vi "Default SubVIs.vi"(8 "error in (no error)":errorcluster, 10 "Unbundler Terminals":refnum<vi>[](array[refnum]), 11 "VI in":refnum<vi>) -> (0 "error out":errorcluster, 2 "SubVI Outputs":refnum<vi>[](array[refnum]), 3 "VI":refnum<vi>)   [LabVIEW 2020, in "Conditum-Tools.lvlib" / "Entity Editor.lvclass"]
uses:
  Entity Editor.lvclass
  <vilib>/Utility/traverseref.llb/TRef TravTarget.ctl
  <vilib>/Utility/miscctls.llb/LVPositionTypeDef.ctl
  <vilib>/IlluminatedG/IG Conditum Base/Conditum/Columns/Type/Set Default.vi
  <vilib>/Utility/traverseref.llb/VI Scripting - Traverse.lvlib
  <vilib>/IlluminatedG/IG Conditum Base/Conditum/Columns/Type/Type.lvclass
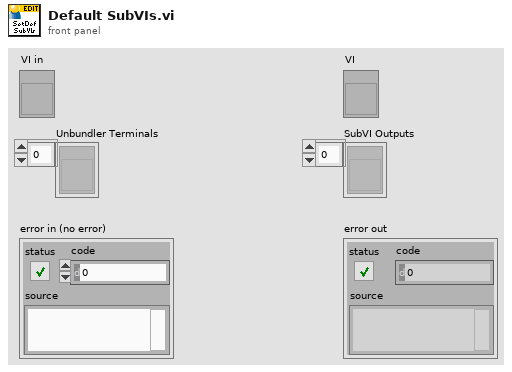
[diagram p1: front panel]
types:
  T1 = typedef "LVPositionTypeDef.ctl" = cluster{"Left":i32, "Top":i32}
  T2 = typedef "TRef TravTarget.ctl" = enum16{"FP", "BD", "Other"}
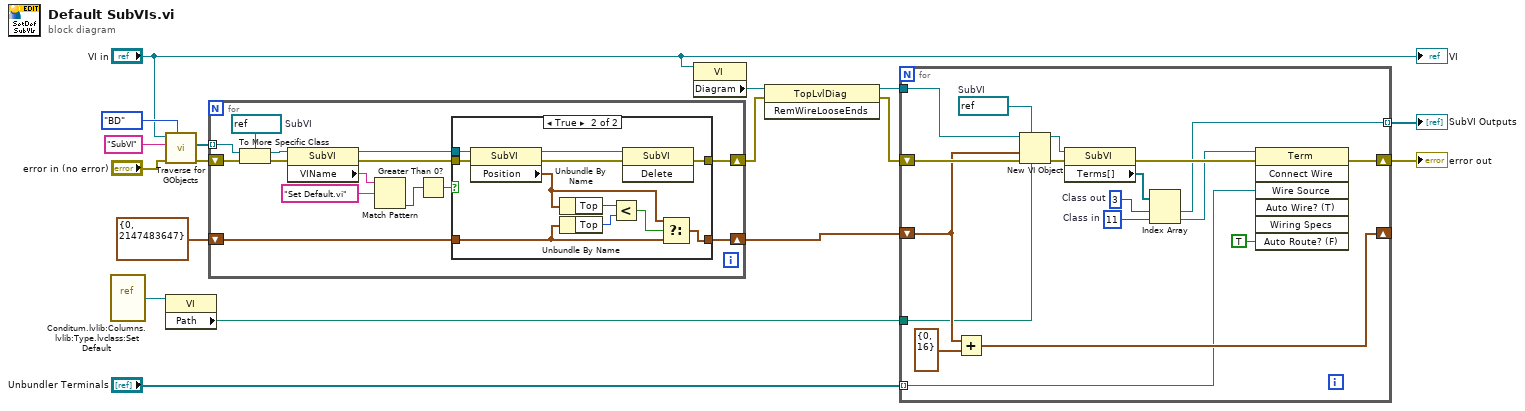
[diagram p0: block diagram]
diagram:
  n1 = vi-ref "Conditum.lvlib:Columns.lvlib:Type.lvclass:Set Default.vi"() -> (w14:refnum<vi>)
  n2 = call <vilib>:"Traverse for GObjects.vi"("Traverse Target"=TRef_TravTarget."BD", "error in (no error)"="error in (no error)", "Class Name"="SubVI", "VI Refnum"="VI in") -> ("error out"=w7:errorcluster, "References"=w8:refnum<vi>[])  [unwired: 4 in, 2 out]
  n3 = property class="VI"(reference=w14) -> ("Path"=w12:path)  [unwired: 1 in, 2 out]
  n4 = for {
    tunnel: w8 -> [w29] mode=indexing
    shift-right: [w31] -> w3
    shift-left: w7 -> [w30]
    shift-right: [w18] -> w1
    shift-left: T1 {"Left"=0, "Top"=2147483647} ("Position") -> [w19]
    w28 = refnum<vi> refnum  # SubVI
    n5 = To More Specific Class(target class=w28, reference=w29, error in=w30) -> (specific class reference=w27:refnum<vi>, error out=w26:errorcluster)
    n6 = property class="SubVI"(reference=w27, error in=w26) -> (reference out=w21:refnum<vi>, error out=w20:errorcluster, "VIName"=w25:string)
    n7 = Match Pattern(string=w25, regular expression="Set Default.vi") -> (offset past match=w23:i32)  [unwired: 1 in, 3 out]
    n8 = Greater Than 0?(x=w23) -> (x > 0?=w22:bool)
    n9 = case shown="True" w22 {
      tunnel: [w33 w44] -> w31
      tunnel: w21 -> [_ w43]
      tunnel: w20 -> [w33 w42]
      tunnel: w19 -> [w32 w37]
      tunnel: [w32 w34] -> w18
      frame False {
      }
      frame True {
        n10 = property class="SubVI"(reference=w43, error in=w42) -> (reference out=w41:refnum<vi>, error out=w40:errorcluster, "Position"=w36:T1)
        n11 = Unbundle By Name(w36) -> ("Top"=w39:i32)
        n12 = Unbundle By Name(w37) -> ("Top"=w38:i32)
        n13 = Less?(x=w39, y=w38) -> (x < y?=w35:bool)
        n14 = invoke class="SubVI" method="Delete"(reference=w41, error in=w40) -> (error out=w44:errorcluster)  [unwired: 1 in, 2 out]
        n15 = Select(t=w36, s=w35, f=w37) -> (s? t:f=w34:T1)
      }
    }
  }
  n16 = property class="VI"(reference="VI in") -> ("Diagram"=w5:refnum<vi>)  [unwired: 1 in, 2 out]
  n17 = invoke class="TopLvlDiag" method="RemWireLooseEnds"(reference=w5, error in=w3) -> (reference out=w4:refnum<vi>, error out=w2:errorcluster)  [unwired: 1 in, 1 out]
  n18 = for {
    tunnel: w4 -> [w59]
    shift-right: [w45] -> w9
    shift-left: w2 -> [w58]
    tunnel: w12 -> [w55]
    shift-right: [w60] -> _
    shift-left: w1 -> [w57]
    tunnel: "Unbundler Terminals" -> [w47] mode=indexing
    tunnel: [w49] -> w10 mode=indexing
    w50 = 3  # Class out
    w51 = 11  # Class in
    w56 = refnum<vi> refnum  # SubVI
    n19 = Add(x=w57, y=T1 {"Left"=0, "Top"=16} ("Position")) -> (x+y=w60:T1)
    n20 = New VI Object(vi object class=w56, owner refnum=w59, position/next to=w57, 6:w55, 8:w58) -> (object refnum=w53:refnum<vi>, 0:w54:errorcluster)  [unwired: 3 in]
    n21 = property class="SubVI"(reference=w53, error in=w54) -> (error out=w62:errorcluster, "Terms[]"=w52:refnum<vi>[])  [unwired: 1 out]
    n22 = Index Array(array=w52, index #1=w50, index #2=w51) -> (element #1=w49:refnum<vi>, element #2=w48:refnum<vi>)
    n23 = invoke class="Term" method="Connect Wire"(reference=w48, error in=w62, "Wire Source"=w47, "Auto Route? (F)"=TRUE) -> (error out=w45:errorcluster)  [unwired: 3 in, 6 out]
  }
  "error out" <- w9
  "SubVI Outputs" <- w10
  "VI" <- "VI in"
